vi "generate_test_file.vi"() -> ()   [LabVIEW 2015]
uses:
  <vilib>/Platform/storage/lvStorage.llb/_openFunction.ctl
  <vilib>/Platform/storage/Storage.llb/usiSequenceRepresentation.ctl
  <vilib>/Platform/storage/Storage.llb/usiOverwriteOptions.ctl
  <vilib>/Platform/storage/lvStorage.llb/_defaultFilePath.vi
  <vilib>/Platform/storage/lvStorage.llb/_openStorageWithRootAutoDetect.vi
  <vilib>/Platform/storage/lvStorage.llb/xStorage/xStorageSupp/ErrorOut.vi
  <vilib>/Platform/storage/Storage.llb/_createExplicitChildObject.vi
  <vilib>/Platform/storage/Storage.llb/__savePropString.vi
  <vilib>/Platform/storage/lvStorage.llb/_saveFloat64Channel.vi
  <vilib>/Platform/storage/lvStorage.llb/_saveInt32Channel.vi
  <vilib>/Platform/storage/lvStorage.llb/__saveInt32Channel.vi
  <vilib>/Platform/storage/Storage.llb/Get Object Info.vi
  <vilib>/Platform/storage/Storage.llb/__closeStorageFromObject.vi
  <vilib>/Platform/storage/lvStorage.llb/xStorage/Open Data Storage/Open Data Storage.xnode
  <vilib>/Platform/storage/lvStorage.llb/xStorage/Write Data/Write Data.xnode
  <vilib>/Platform/storage/lvStorage.llb/xStorage/Close Data Storage/Close Data Storage.xnode
panel:
  out "error out":errorcluster
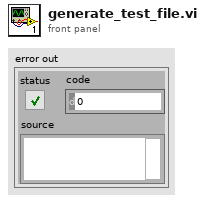
[diagram p1: front panel]
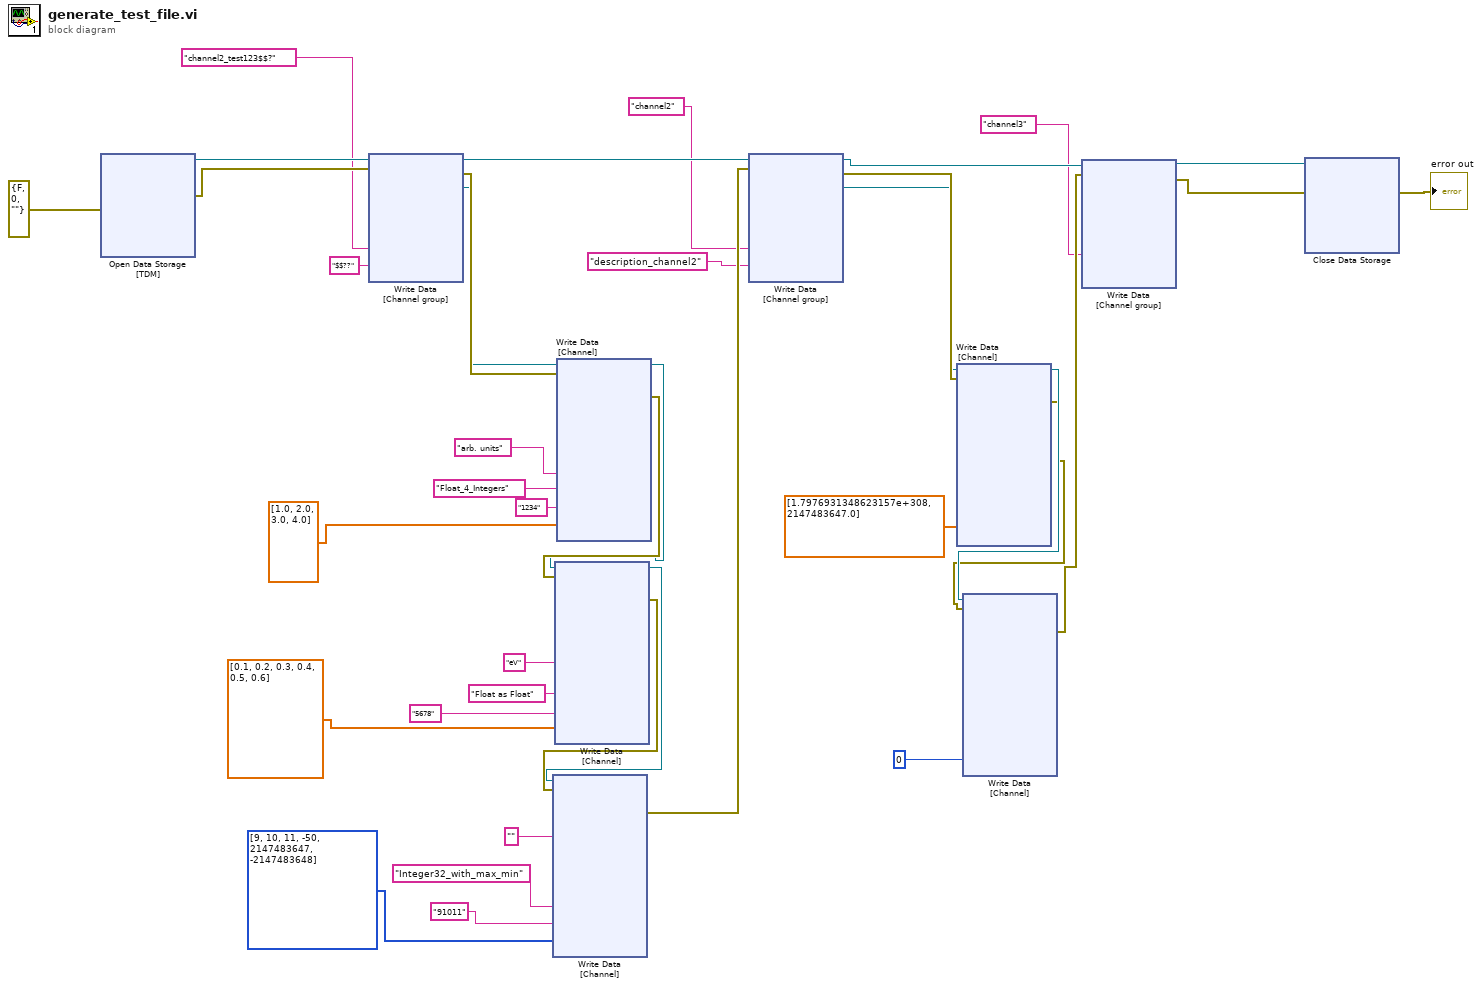
[diagram p0: block diagram]
diagram:
  n1 = xnode "Open Data Storage\n[TDM]"("error in (no error)"=errorcluster {"status"=FALSE, "code"=0, "source"=""}) -> ("storage refnum (file)"=w37:refnum<k20>, "error out"=w38:errorcluster)  [unwired: 4 in, 1 out]
  n2 = xnode "Write Data\n[Channel group]"("Name"="channel2_test123$$?", "Description"="$$??", "storage refnum (file)"=w37, "error in"=w38) -> ("storage refnum (file) out"=w7:refnum<k20>, "error out"=w33:errorcluster, "storage refnum (channel group)"=w8:refnum<k20>)
  n3 = xnode "Write Data\n[Channel]"("Unit"="arb. units", "Name"="Float_4_Integers", "Description"="1234", "Signal"=dbl[] [1.0, 2.0, 3.0, 4.0], "storage refnum (channel group)"=w8, "error in"=w33) -> ("storage refnum (channel group) out"=w30:refnum<k20>, "error out"=w32:errorcluster)  [unwired: 2 in, 1 out]
  n4 = xnode "Write Data\n[Channel]"("Unit"="eV", "Name"="Float as Float", "Description"="5678", "Signal"=dbl[] [0.1, 0.2, 0.3, 0.4, 0.5, 0.6], "storage refnum (channel group)"=w30, "error in"=w32) -> ("storage refnum (channel group) out"=w29:refnum<k20>, "error out"=w31:errorcluster)  [unwired: 2 in, 1 out]
  n5 = xnode "Write Data\n[Channel]"("Unit"="", "Name"="Integer32_with_max_min", "Description"="91011", "Signal"=i32[] [9, 10, 11, -50, 2147483647, -2147483648], "storage refnum (channel group)"=w29, "error in"=w31) -> ("error out"=w28:errorcluster)  [unwired: 2 in, 2 out]
  n6 = xnode "Write Data\n[Channel group]"("Name"="channel2", "Description"="description_channel2", "storage refnum (file)"=w7, "error in"=w28) -> ("storage refnum (file) out"=w4:refnum<k20>, "error out"=w14:errorcluster, "storage refnum (channel group)"=w5:refnum<k20>)
  n7 = xnode "Write Data\n[Channel]"("Signal"=dbl[] [1.7976931348623157e+308, 2147483647.0], "storage refnum (channel group)"=w5, "error in"=w14) -> ("storage refnum (channel group) out"=w12:refnum<k20>, "error out"=w11:errorcluster)  [unwired: 5 in, 1 out]
  n8 = xnode "Write Data\n[Channel]"("Signal"=0, "storage refnum (channel group)"=w12, "error in"=w11) -> ("error out"=w10:errorcluster)  [unwired: 5 in, 2 out]
  n9 = xnode "Write Data\n[Channel group]"("Name"="channel3", "storage refnum (file)"=w4, "error in"=w10) -> ("storage refnum (file) out"=w36:refnum<k20>, "error out"=w35:errorcluster)  [unwired: 1 in, 1 out]
  n10 = xnode "Close Data Storage\n"("storage refnum (file)"=w36, "error in (no error)"=w35) -> ("error out"=→"error out":errorcluster)  [unwired: 1 out]
